vi "VI Tree.vi"   [LabVIEW 2011, in "Fluke 8508.lvlib"]
doc: "This is the instrument driver for the fl8508a Reference Multimeter. The VI Tree displays all the user-callable VIs of the instrument driver in an organized table."
uses:
  Fluke 8508.lvlib
  Configure/Configure Normal Resistance.vi
  Configure/Temperature VIs/Configure ITS90 Conversion.vi
panel:
  # "© 2005 National Instruments.  ALL RIGHTS RESERVED."
  # "SEE DIAGRAM\nFOR VI TREE."
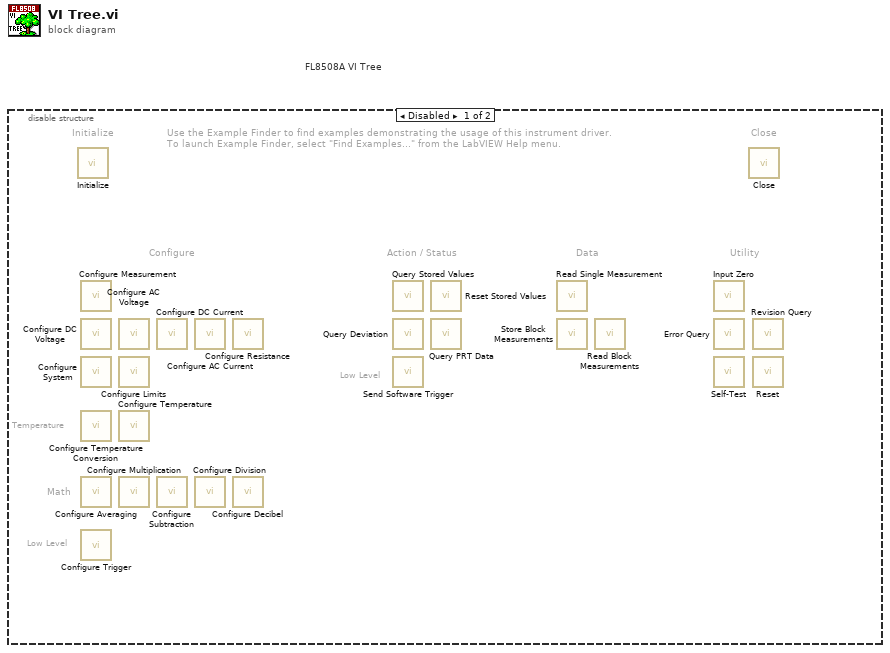
[diagram p0: block diagram]
diagram:
  # "FL8508A VI Tree"
  n1 = disable-structure shown="Disabled" {
    frame Disabled {
      # "Temperature"
      # "Math"
      # "Action / Status"
      # "Low Level"
      # "Low Level"
      # "Use the Example Finder to find examples demonstrating the usage of this instrument driver.\nTo launch Example Finder, select \"Find Examples...\" from the LabVIEW Help menu."
      # "Configure"
      # "Utility"
      # "Data"
      # "Close"
      # "Initialize"
      n2 = call "Initialize.vi"() -> ()  [unwired: 10 in, 2 out]
      n3 = call "Configure Measurement.vi"() -> ()  [unwired: 10 in, 2 out]
      n4 = call "Configure DC Voltage.vi"() -> ()  [unwired: 10 in, 2 out]
      n5 = call "Configure System.vi"() -> ()  [unwired: 10 in, 2 out]
      n6 = call-poly "Configure Temperature Conversion.vi"() -> ()  [unwired: 14 in, 2 out]
      n7 = call "Configure Averaging.vi"() -> ()  [unwired: 10 in, 2 out]
      n8 = call "Configure Trigger.vi"() -> ()  [unwired: 10 in, 2 out]
      n9 = call "Configure AC Voltage.vi"() -> ()  [unwired: 14 in, 2 out]
      n10 = call "Configure Limits.vi"() -> ()  [unwired: 10 in, 2 out]
      n11 = call "Configure Temperature.vi"() -> ()  [unwired: 10 in, 2 out]
      n12 = call "Configure Multiplication.vi"() -> ()  [unwired: 10 in, 2 out]
      n13 = call "Configure DC Current.vi"() -> ()  [unwired: 10 in, 2 out]
      n14 = call "Configure Subtraction.vi"() -> ()  [unwired: 10 in, 2 out]
      n15 = call "Configure AC Current.vi"() -> ()  [unwired: 10 in, 2 out]
      n16 = call "Configure Division.vi"() -> ()  [unwired: 10 in, 2 out]
      n17 = call-poly "Configure Resistance.vi"() -> ()  [unwired: 10 in, 2 out]
      n18 = call "Configure Decibel.vi"() -> ()  [unwired: 10 in, 2 out]
      n19 = call "Query Stored Values.vi"() -> ()  [unwired: 6 in, 6 out]
      n20 = call "Query Deviation.vi"() -> ()  [unwired: 9 in, 3 out]
      n21 = call "Send Software Trigger.vi"() -> ()  [unwired: 10 in, 2 out]
      n22 = call "Reset Stored Values.vi"() -> ()  [unwired: 10 in, 2 out]
      n23 = call "Query PRT Data.vi"() -> ()  [unwired: 9 in, 3 out]
      n24 = call "Read Single Measurement.vi"() -> ()  [unwired: 9 in, 3 out]
      n25 = call "Store Block Measurements.vi"() -> ()  [unwired: 10 in, 2 out]
      n26 = call "Read Block Measurements.vi"() -> ()  [unwired: 9 in, 3 out]
      n27 = call "Input Zero.vi"() -> ()  [unwired: 9 in, 3 out]
      n28 = call "Error Query.vi"() -> ()  [unwired: 8 in, 4 out]
      n29 = call "Self-Test.vi"() -> ()  [unwired: 9 in, 3 out]
      n30 = call "Close.vi"() -> ()  [unwired: 11 in, 1 out]
      n31 = call "Revision Query.vi"() -> ()  [unwired: 8 in, 4 out]
      n32 = call "Reset.vi"() -> ()  [unwired: 10 in, 2 out]
    }
    frame Enabled {
    }
  }
